vi "Parse Queue Service Properties.vi"(11 "Queue service string":string) -> (3 "Queue service properties":T1)   [LabVIEW 2015, in "NI_Azure_Queue.lvlib"]
uses:
  NI_Azure_Queue.lvlib
  Queue Service Properties.ctl
  Logging.ctl
  Retention Policy.ctl
  Metrics.ctl
  Cors Rule.ctl
  XML Parsing/NI_Azure_XML Parsing.lvlib
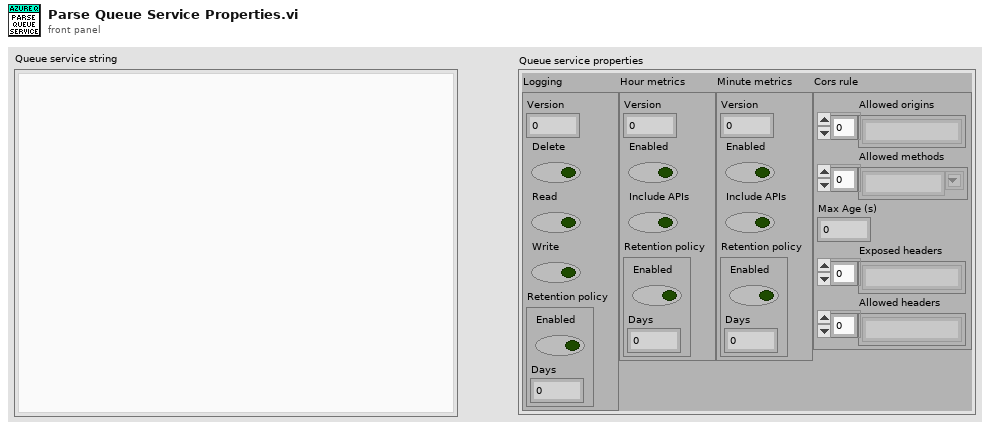
[diagram p1: front panel]
types:
  T1 = typedef "NI_Azure_Queue.lvlib/Queue Service Properties.ctl" = cluster{"Logging":T2, "Hour metrics":T4, "Minute metrics":T4, "Cors rule":T5}
  T2 = typedef "NI_Azure_Queue.lvlib/Logging.ctl" = cluster{"Version":dbl, "Delete":bool, "Read":bool, "Write":bool, "Retention policy":T3}
  T3 = typedef "NI_Azure_Queue.lvlib/Retention Policy.ctl" = cluster{"Enabled":bool, "Days":u32}
  T4 = typedef "NI_Azure_Queue.lvlib/Metrics.ctl" = cluster{"Version":dbl, "Enabled":bool, "Include APIs":bool, "Retention policy":T3}
  T5 = typedef "NI_Azure_Queue.lvlib/Cors Rule.ctl" = cluster{"Allowed origins":string[], "Allowed methods":string[], "Max Age (s)":u32, "Exposed headers":string[], "Allowed headers":string[]}
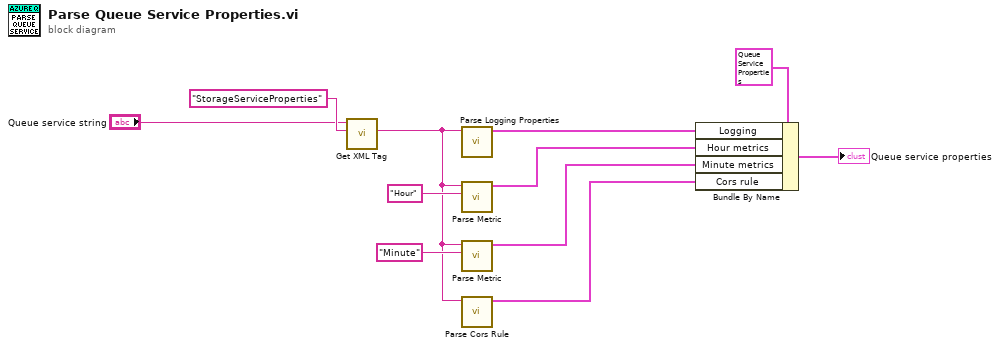
[diagram p0: block diagram]
diagram:
  n1 = call "Get XML Tag.vi"("Tag name"="StorageServiceProperties", "XML String in"="Queue service string") -> ("Tag value"=w2:string)  [unwired: 5 in, 4 out]
  n2 = call "Parse Logging Properties.vi"("String"=w2) -> ("Logging properties"=w8:T2)  [unwired: 10 in]
  n3 = call "Parse Metric.vi"("Metric name"="Hour", "String"=w2) -> ("Metric properties"=w6:T4)  [unwired: 9 in]
  n4 = call "Parse Metric.vi"("Metric name"="Minute", "String"=w2) -> ("Metric properties"=w4:T4)  [unwired: 9 in]
  n5 = call "Parse Cors Rule.vi"("String"=w2) -> ("Cors rule"=w3:T5)  [unwired: 10 in]
  n6 = Bundle By Name(cluster=T1 {"Logging"={"Version"=0.0, "Delete"=FALSE, "Read"=FALSE, "Write"=FALSE, "Retention policy"={"Enabled"=FALSE, "Days"=0}}, "Hour metrics"={"Version"=0.0, "Enabled"=FALSE, "Include APIs"=FALSE, "Retention policy"={"Enabled"=FALSE, "Days"=0}}, "Minute metrics"={"Version"=0.0, "Enabled"=FALSE, "Include APIs"=FALSE, "Retention policy"={"Enabled"=FALSE, "Days"=0}}, "Cors rule"={"Allowed origins"=[], "Allowed methods"=[], "Max Age (s)"=0, "Exposed headers"=[], "Allowed headers"=[]}} ("Blob service properties"), "Logging"=w8, "Hour metrics"=w6, "Minute metrics"=w4, "Cors rule"=w3) -> (→"Queue service properties":T1)
